vi "tsdb_get_flexray_db_properties_by_address_verbose.vi"(8 "error in (no error)":errorcluster caption="错误输入（无错误）", 10 "AAddr":string, 11 "path in":path) -> (0 "error out":errorcluster caption="错误输出", 1 "flexray_db_properties":T1, 2 "function return":i32, 3 "path out":path)   [LabVIEW 2014]
doc: "Call location\nInput parameter AAddd: database address\nADBIndex：\n Returned database index\nASignalCount：\n Number of returned signals\nAFrameCount：\n Number of returned messages\nAECUCount：\n Number of returned ECUs\nASupportedChannelMask：\n Returned support channel mask\nAName：\n Database Name\nAComment：\n notes\nReturn value 0: Successful execution\nOther values: Failed"
uses:
  Typedef/FlexRay/flexray_db_properties.ctl
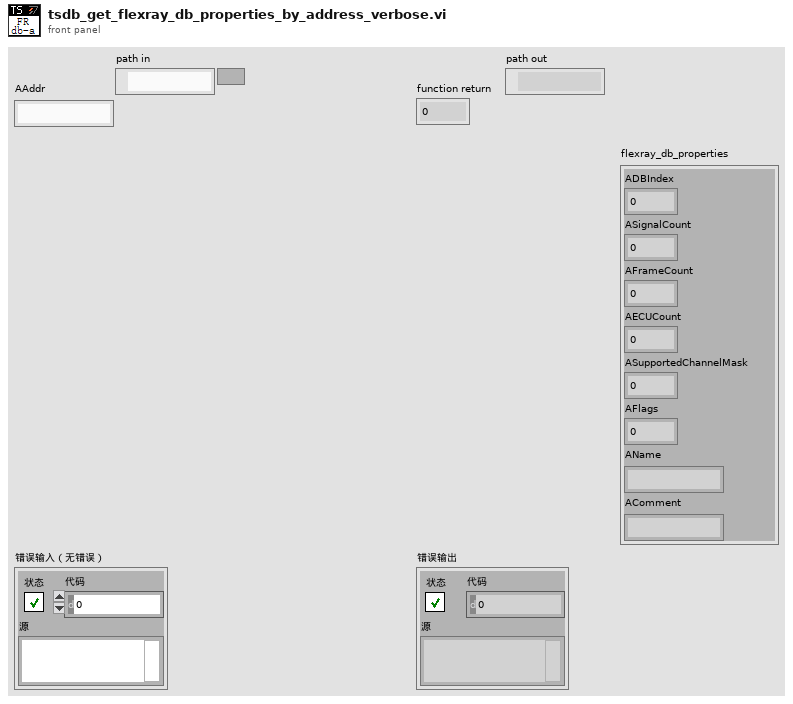
[diagram p1: front panel]
types:
  T1 = typedef "flexray_db_properties.ctl" = cluster{"ADBIndex":i32, "ASignalCount":i32, "AFrameCount":i32, "AECUCount":i32, "ASupportedChannelMask":i64, "AFlags":i64, "AName":string, "AComment":string}
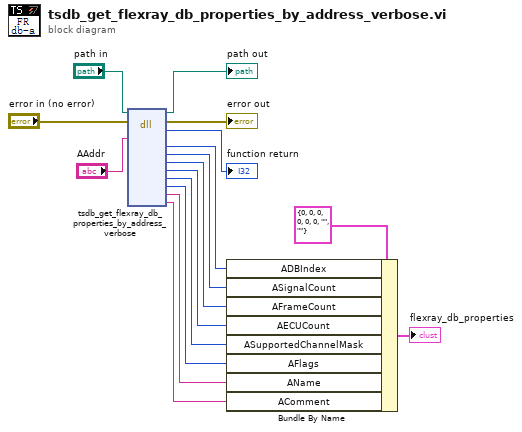
[diagram p0: block diagram]
diagram:
  n1 = dll-call lib="D:/Work/LabVIEW Code/TSMaster Labview SDK/LabVIEW/LabVIEW-TSMasterAPI_CLN/TSMasterAPI_LabVIEW-2024-10-08 14-20-13/Not_organized_vi/TSMaster.*" fn="tsdb_get_flexray_db_properties_by_address_verbose"(path in="path in", error in="error in (no error)", "AAddr"="AAddr") -> (path out=→"path out":path, error out=→"error out":errorcluster, "返回类型"=→"function return":i32, "ADBIndex"=w8:i32, "ASignalCount"=w7:i32, "AFrameCount"=w6:i32, "AECUCount"=w5:i32, "ASupportedChannelMask"=w4:i64, "AFlags"=w3:i64, "AName"=w2:string, "AComment"=w1:string)  [unwired: 10 in]
  n2 = Bundle By Name(cluster=T1 {"ADBIndex"=0, "ASignalCount"=0, "AFrameCount"=0, "AECUCount"=0, "ASupportedChannelMask"=0, "AFlags"=0, "AName"="", "AComment"=""} ("flexray_db_properties"), "ADBIndex"=w8, "ASignalCount"=w7, "AFrameCount"=w6, "AECUCount"=w5, "ASupportedChannelMask"=w4, "AFlags"=w3, "AName"=w2, "AComment"=w1) -> (→"flexray_db_properties":T1)
